vi "ADCMT7451A Read Memory Data ADC.vi"() -> ()   [LabVIEW 2017]
doc: "This example shows how to configure a measurement, set up triggering, trigger a measurement, and retrieve a measurement. It shows how to use the low-level Data VIs to retrieve data from the DMM."
uses:
  Public/Configure/Configure DC Volts.vi
  Public/Configure/Configure 2W Resistance.vi
  Public/Configure/Configure DC Current.vi
  ADCMT7451_ADC.lvlib
panel:
  in  "Manual Range (0)":dbl=1.0 format="%#.6p"
  out "Measurements":dbl[](array[numeric])
  in  "Sample Count (100)":i32=100 min=1 max=16000 format="%#.6g"
  out "Waveform Chart":dbl[](graph)
  in  "Function (0: DC Volts)":u16(ring) items=["DC Volts", "2-Wire Resistance", "DC Current"]
  in  "VISA resource name":refnum<visa-resource-name>
  # "(c) 2008 ADCMT ADC Corporation.  ALL RIGHTS RESERVED."
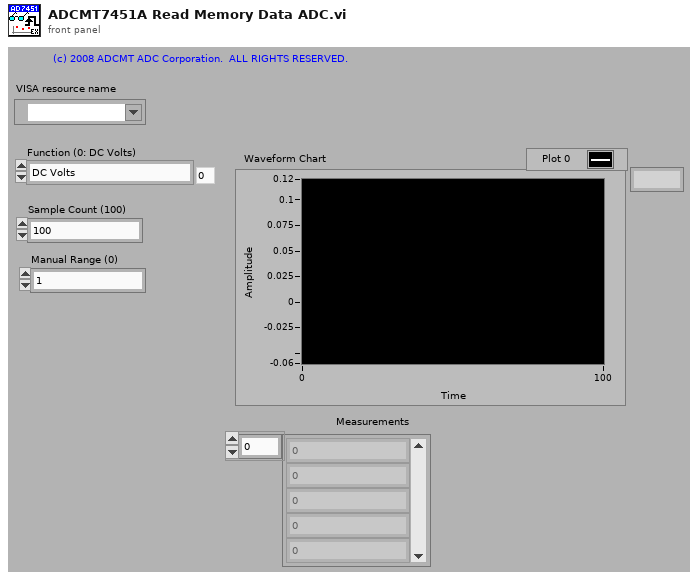
[diagram p1: front panel]
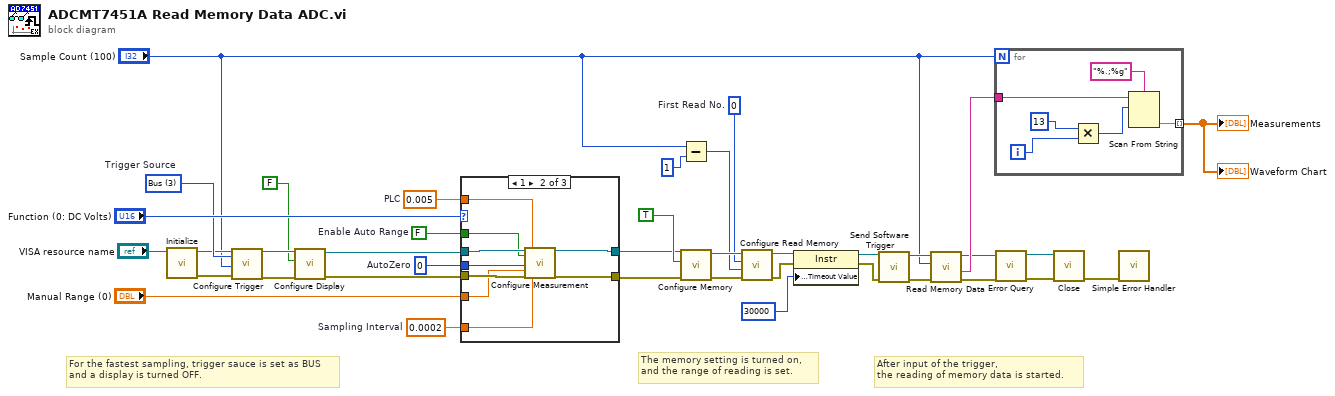
[diagram p0: block diagram]
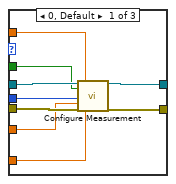
[diagram p2: hidden frame]
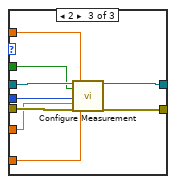
[diagram p3: hidden frame]
diagram:
  w15 = 0  # First Read No.
  w22 = u16 3 items=["Immediate", "Manual", "External", "Bus"]  # Trigger Source
  w30 = 0.005  # PLC
  w28 = 0.0002  # Sampling Interval
  w31 = 0  # AutoZero
  w32 = FALSE  # Enable Auto Range
  # "The memory setting is turned on, \nand the range of reading is set."
  # "After input of the trigger,\nthe reading of memory data is started."
  # "For the fastest sampling, trigger sauce is set as BUS \nand a display is turned OFF."
  n1 = call "Initialize.vi"("VISA resource name"="VISA resource name") -> ("error out"=w21:errorcluster, "VISA resource name out"=w20:refnum<visa-resource-name>)  [unwired: 9 in]
  n2 = call "Configure Trigger.vi"("VISA resource name"=w20, "Trigger Source (0: Immediate)"=w22, "Sample Count (1)"="Sample Count (100)", "error in (no error)"=w21) -> ("VISA resource name out"=w10:refnum<visa-resource-name>, "error out"=w11:errorcluster)  [unwired: 14 in]
  n3 = call "Configure Display.vi"("error in (no error)"=w11, "Display (T: On)"=FALSE, "VISA resource name"=w10) -> ("error out"=w8:errorcluster, "VISA resource name out"=w9:refnum<visa-resource-name>)  [unwired: 7 in]
  n4 = case shown="1" "Function (0: DC Volts)" {
    tunnel: w9 -> [w47 w56 w63]
    tunnel: [w44 w55 w64] -> w18
    tunnel: [w45 w54 w65] -> w19
    tunnel: w8 -> [w46 w53 w62]
    tunnel: w32 -> [w43 w50 w59]
    tunnel: w31 -> [w42 w51 w60]
    tunnel: w30 -> [w41 w49 w58]
    tunnel: w28 -> [w40 w52 w61]
    tunnel: "Manual Range (0)" -> [w39 w48 w57]
    frame 0, Default {
      n5 = call-poly "Configure Measurement.vi"("VISA resource name"=w47, "Enable Auto Range (T:Enable)"=w43, "Auto-zero (1: On)"=w42, "Manual Range (0 V)"=w39, "error in (no error)"=w46, "Power Line Cycles (1.00)"=w41, "Sampling Interval (0.05)"=w40) -> ("VISA resource name out"=w44:refnum<visa-resource-name>, "error out"=w45:errorcluster)  [unwired: 11 in]
    }
    frame 1 {
      n6 = call-poly "Configure Measurement.vi"("VISA resource name"=w56, "Enable Auto Range (T: Enable)"=w50, "Auto-zero (1: On)"=w51, "Manual Range (0 Ohm)"=w48, "error in (no error)"=w53, "Power Line Cycles (1.00)"=w49, "Sampling Interval (0.05s)"=w52) -> ("VISA resource name out"=w55:refnum<visa-resource-name>, "error out"=w54:errorcluster)  [unwired: 11 in]
    }
    frame 2 {
      n7 = call-poly "Configure Measurement.vi"("VISA resource name"=w63, "Enable Auto Range (T: Enable)"=w59, "Auto-zero (1: On)"=w60, "Manual Range (0 A)"=w57, "error in (no error)"=w62, "Power Line Cycles (1.00)"=w58, "Sampling Interval (0.05)"=w61) -> ("VISA resource name out"=w64:refnum<visa-resource-name>, "error out"=w65:errorcluster)  [unwired: 11 in]
    }
  }
  n8 = Subtract(x="Sample Count (100)", y=1) -> (x-y=w14:i32)
  n9 = call "Configure Memory.vi"("error in (no error)"=w19, "Store (T: On)"=TRUE, "VISA resource name"=w18) -> ("error out"=w17:errorcluster, "VISA resource name out"=w16:refnum<visa-resource-name>)  [unwired: 7 in]
  n10 = call "Configure Read Memory.vi"("error in (no error)"=w17, "Last Read No."=w14, "First Read No."=w15, "VISA resource name"=w16) -> ("error out"=w3:errorcluster, "VISA resource name out"=w4:refnum<visa-resource-name>)  [unwired: 5 in, 1 out]
  n11 = property class="Instr"(reference=w4, error in=w3, "General Settings:Timeout Value"=u32 30000) -> (reference out=w2:refnum<visa-resource-name>, error out=w1:errorcluster)
  n12 = call "Send Software Trigger.vi"("error in (no error)"=w1, "VISA resource name"=w2) -> ("error out"=w26:errorcluster, "VISA resource name out"=w27:refnum<visa-resource-name>)  [unwired: 8 in]
  n13 = call "Read Memory Data.vi"("error in (no error)"=w26, "Read Count (1)"="Sample Count (100)", "VISA resource name"=w27) -> ("error out"=w23:errorcluster, "Measurements"=w25:string, "VISA resource name out"=w24:refnum<visa-resource-name>)  [unwired: 6 in]
  n14 = for {
    N: "Sample Count (100)" -> [_]
    tunnel: [w71] -> w34 mode=indexing
    tunnel: w25 -> [w69]
    i -> [w67]
    n15 = Multiply(x=13, y=w67) -> (x*y=w66:i32)
    n16 = Scan From String(format string="%.;%g", input string=w69, initial scan location=w66) -> (output 1=w71:dbl)  [unwired: 2 in, 3 out]
  }
  "Measurements" <- w34
  "Waveform Chart" <- w34
  n17 = call "Error Query.vi"("error in (no error)"=w23, "VISA resource name"=w24) -> ("error out"=w35:errorcluster, "VISA resource name out"=w36:refnum<visa-resource-name>)  [unwired: 6 in, 2 out]
  n18 = call "Close.vi"("error in (no error)"=w35, "VISA resource name"=w36) -> ("error out"=w37:errorcluster)  [unwired: 9 in]
  n19 = call <vilib>:"Simple Error Handler.vi"("error in (no error)"=w37) -> ()  [unwired: 4 in, 5 out]
